vi "Get Setting - Error_Log_Setting.vi"(8 "Error In":errorcluster) -> (0 "Error Out":errorcluster, 3 "Error_Log_Setting":T1)   [LabVIEW 2016, in "Error Manager.lvlib" / "Settings.lvclass"]
uses:
  Settings.lvclass
  Settings (class variable).vi
  Error_Log_Setting (enum).ctl
panel:
  # "Input\nInputs to the VI"
  # "Development\nControls or indicators that are useful for development or testing, but which are not outputs of the VI."
  # "Output\nOutputs of the VI"
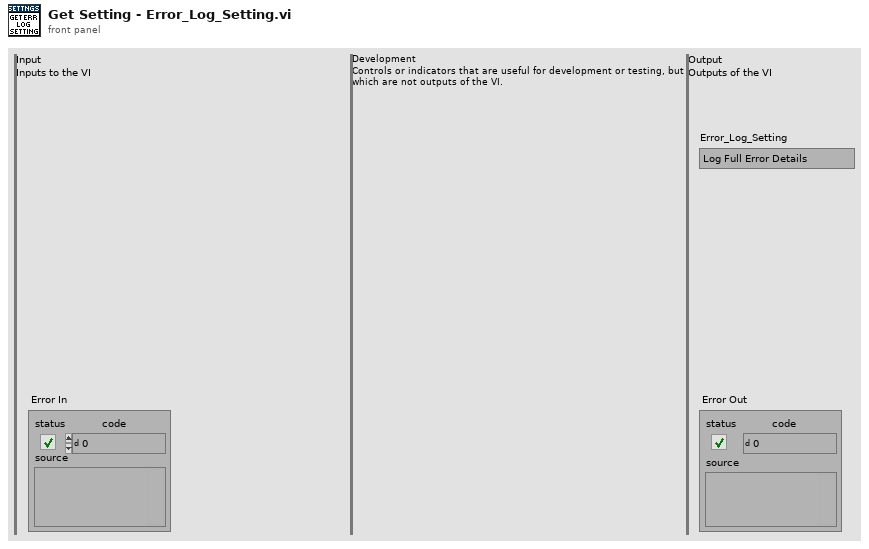
[diagram p1: front panel]
types:
  T1 = typedef "Error Manager.lvlib/Settings.lvclass/Error_Log_Setting (enum).ctl" = enum16{"Log Full Error Details", "Log Error Codes Only", "Do Not Log"}
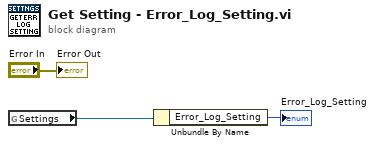
[diagram p0: block diagram]
diagram:
  n1 = global read "Settings (class variable).vi" "Settings"() -> (w1:refnum<class "Settings.lvclass">)
  n2 = Unbundle By Name(w1) -> ("Error_Log_Setting"=→"Error_Log_Setting":T1)
  "Error Out" <- "Error In"
